vi "Close AO.vi"(8 "error in (no error)":errorcluster, 11 "AO in":T1) -> (0 "error out":errorcluster)   [LabVIEW 2019, in "Inputs.lvlib"]
uses:
  Inputs.lvlib
  Ctl/AO.ctl
  Ctl/Parameter State.ctl
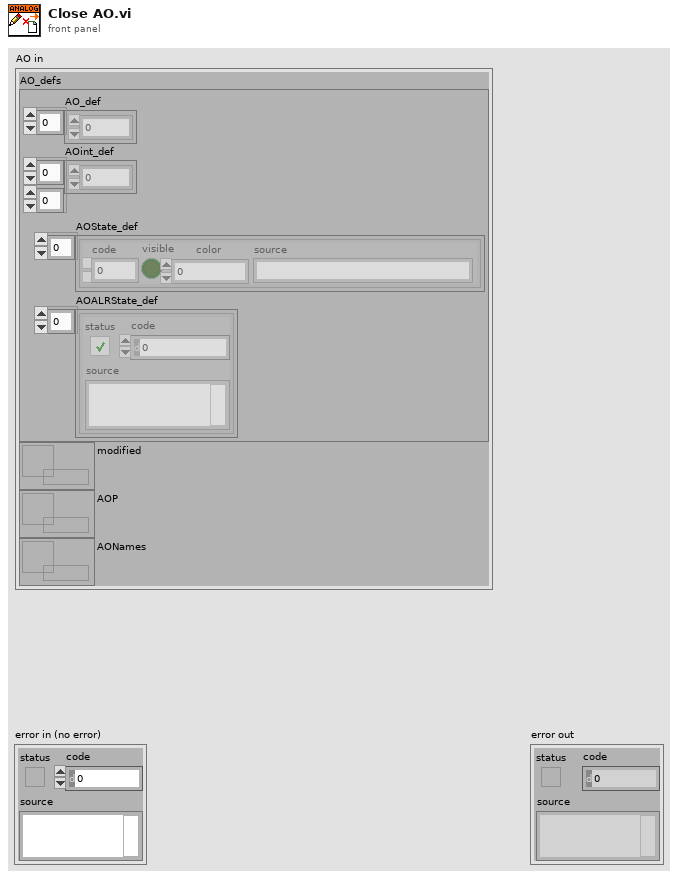
[diagram p1: front panel]
types:
  T1 = typedef "Inputs.lvlib/AO.ctl" = cluster{"AO_defs":cluster{"AO_def":dbl[], "AOint_def":u16[][], "AOState_def":T2[], "AOALRState_def":errorcluster[]}, "modified":refnum<data-value>, "AOP":refnum<data-value>, "AONames":refnum<data-value>}
  T2 = typedef "Inputs.lvlib/Parameter State.ctl" = cluster{"code":i32, "visible":bool, "color":u32, "source":string}
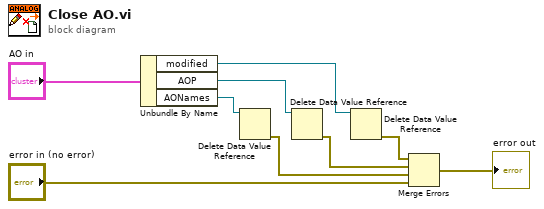
[diagram p0: block diagram]
diagram:
  n1 = Unbundle By Name("AO in") -> ("modified"=w9:refnum<data-value>, "AOP"=w7:refnum<data-value>, "AONames"=w6:refnum<data-value>)
  n2 = Delete Data Value Reference(data value reference=w6) -> (error out=w4:errorcluster)  [unwired: 1 in, 1 out]
  n3 = Delete Data Value Reference(data value reference=w7) -> (error out=w5:errorcluster)  [unwired: 1 in, 1 out]
  n4 = Delete Data Value Reference(data value reference=w9) -> (error out=w8:errorcluster)  [unwired: 1 in, 1 out]
  n5 = Merge Errors(w8, w5, w4, "error in (no error)") -> (→"error out":errorcluster)
